vi "tcs_issueCommand_standby.vi"(8 "error in (no error)":errorcluster, 11 "command_standby_Ctl":T1) -> (0 "error out":errorcluster, 2 "function return":i32, 3 "command_standby_Ctl out":T1)   [LabVIEW 2016, in "SALLV_tcs.lvlib"]
doc: "int tcs_shm_issueCommand_standbyLV(tcs_command_standbyLV *command_standby_Ctl );"
uses:
  SALLV_tcs.lvlib
  DataTypes/command_standby.ctl
  SALLV_tcs.so
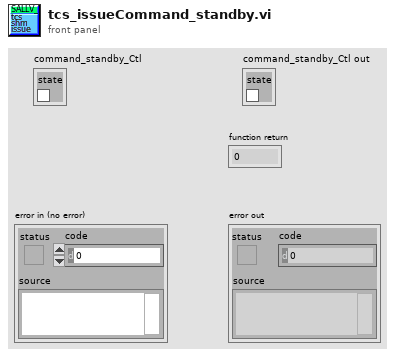
[diagram p1: front panel]
types:
  T1 = typedef "SALLV_tcs.lvlib/command_standby.ctl" = cluster{"state":bool}
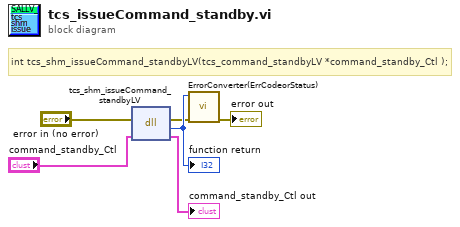
[diagram p0: block diagram]
diagram:
  # "int tcs_shm_issueCommand_standbyLV(tcs_command_standbyLV *command_standby_Ctl );"
  n1 = dll-call lib="home/andres/Desktop/SALLV_tcs/SALLV_tcs.*" fn="tcs_shm_issueCommand_standbyLV"(error in="error in (no error)", "command_standby_Ctl"="command_standby_Ctl") -> (error out=w2:errorcluster, w6:i32, "command_standby_Ctl"=→"command_standby_Ctl out":T1)  [unwired: 2 in, 1 out]
  "function return" <- w6
  n2 = call "ErrorConverter(ErrCodeorStatus).vi"("error in (no error)"=w2, "error code"=w6) -> ("error out"=→"error out":errorcluster)  [unwired: 9 in]
